vi "Ramp Generation.vi"() -> ()   [LabVIEW 2025]
panel:
  out "Ramp Output":waveform(dbl)(graph)
  in  "# Points":dbl
  in  "Max":dbl
  in  "Time Span (s)":dbl
  in  "Min":dbl
  # "ME 235: Design of Microprocessor Based Mechanical Systems"
  # "Lab 2 - Ramp Generation"
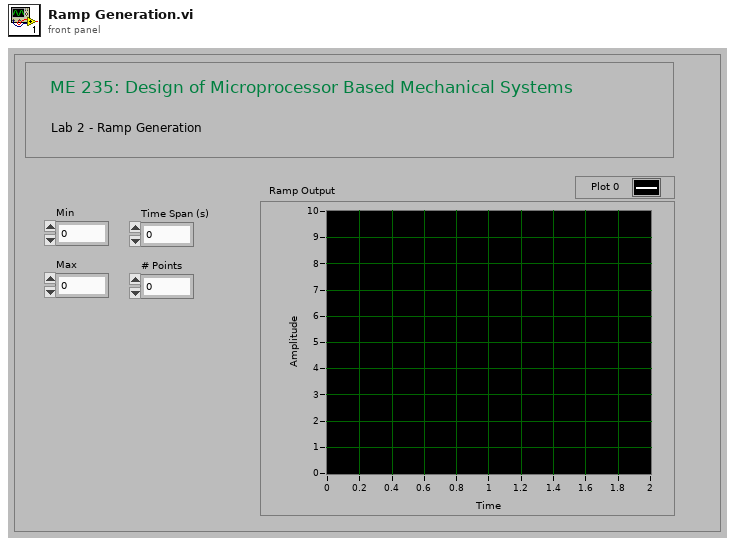
[diagram p1: front panel]
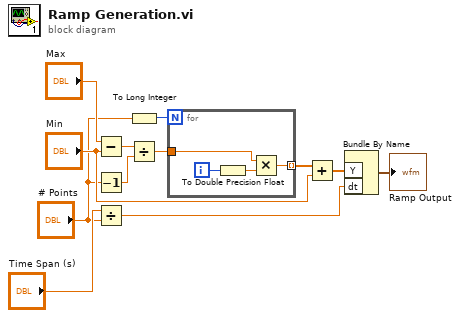
[diagram p0: block diagram]
diagram:
  n1 = Subtract(x="Max", y="Min") -> (x-y=w5:dbl)
  n2 = Decrement(x="# Points") -> (x-1=w8:dbl)
  n3 = Divide(x="Time Span (s)", y="# Points") -> (x/y=w11:dbl)
  n4 = To Long Integer(number="# Points") -> (32bit integer=w2:i32)
  n5 = Divide(x=w5, y=w8) -> (x/y=w4:dbl)
  n6 = for {
    N: w2 -> [_]
    tunnel: w4 -> [w14]
    tunnel: [w13] -> w3 mode=indexing
    i -> [w16]
    n7 = To Double Precision Float(number=w16) -> (double precision float=w15:dbl)
    n8 = Multiply(x=w14, y=w15) -> (x*y=w13:dbl)
  }
  n9 = Add(x=w3, y="Min") -> (x+y=w9:dbl[])
  n10 = Bundle By Name("Y"=w9, "dt"=w11) -> (→"Ramp Output":waveform(dbl))  [unwired: 1 in]
